vi "DSPClearBuffer.vi"(1 "Inst info":T1, 2 "ramp?":bool) -> ()   [LabVIEW 2013]
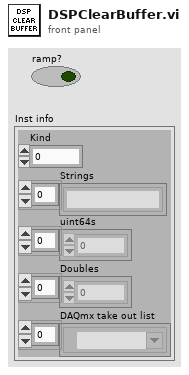
[diagram p1: front panel]
types:
  T1 = cluster{"Kind":u16, "Strings":string[], "uint64s":u64[], "Doubles":dbl[], "DAQmx take out list":refnum<k21>[]}
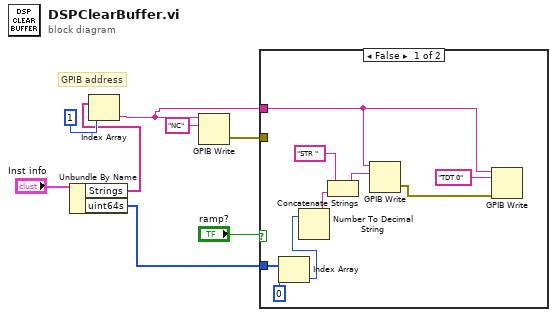
[diagram p0: block diagram]
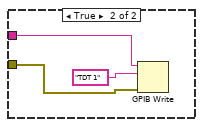
[diagram p2: hidden frame]
diagram:
  # "GPIB address"
  n1 = Unbundle By Name("Inst info") -> ("Strings"=w6:string[], "uint64s"=w2:u64[])
  n2 = Index Array(array=w6, index=1) -> (element=w3:string)
  n3 = GPIB Write(0:w3, 1:"NC") -> (6:w4:errorcluster)  [unwired: 3 in, 1 out]
  n4 = case shown="False" "ramp?" {
    tunnel: w4 -> [_ w19]
    tunnel: w3 -> [w12 w18]
    tunnel: w2 -> [w11 _]
    frame False {
      n5 = Index Array(array=w11, index=0) -> (element=w9:u64)
      n6 = Number To Decimal String(number=w9) -> (decimal integer string=w14:string)  [unwired: 1 in]
      n7 = Concatenate Strings("STR ", w14) -> (w15:string)
      n8 = GPIB Write(0:w12, 1:w15) -> (6:w13:errorcluster)  [unwired: 3 in, 1 out]
      n9 = GPIB Write(0:w12, 1:"TDT 0", 3:w13) -> ()  [unwired: 2 in, 2 out]
    }
    frame True {
      n10 = GPIB Write(0:w18, 1:"TDT 1", 3:w19) -> ()  [unwired: 2 in, 2 out]
    }
  }
